vi "Annotate April.vi"(6 "hilight":bool, 7 "Annotate":bool, 9 "cutoffs":T1, 10 "Detected Tags":T3(array[cluster]), 11 "Refnum in":T2) -> (1 "margins":dbl[](array[numeric]), 2 "tags":T3(array[cluster]), 3 "Refnum out":T2)   [LabVIEW 2023]
uses:
  <vilib>/vision/Image Controls.llb/IMAQ Image.ctl
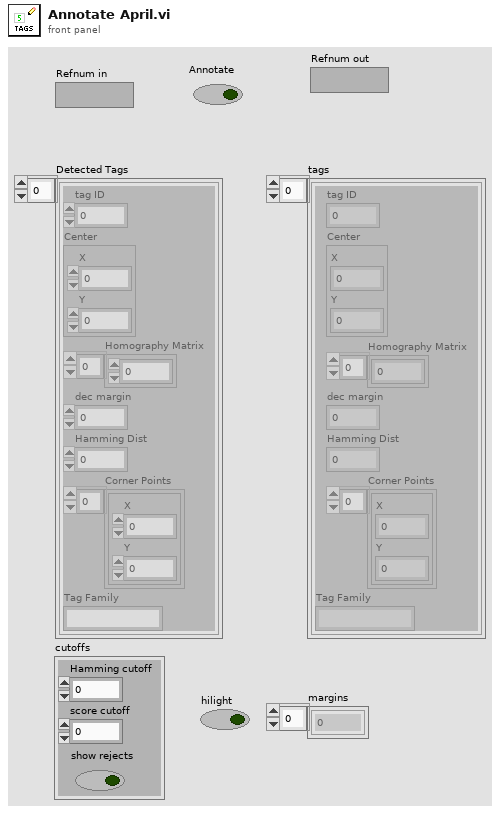
[diagram p1: front panel]
types:
  T1 = cluster{"Hamming cutoff":i32, "score cutoff":dbl, "show rejects":bool}
  T2 = typedef "IMAQ Image.ctl" = refnum<image>
  T3 = cluster{"tag ID":i32, "Center":cluster{"X":dbl, "Y":dbl}, "Homography Matrix":dbl[], "dec margin":dbl, "Hamming Dist":i32, "Corner Points":cluster{"X":dbl, "Y":dbl}[], "Tag Family":string}[]
  T4 = cluster{"Desired Font (Application)":enum16{"User-specified Font", "Application Font", "System Font", "Dialog Font"}, "[User-specified Font]":cluster{"Font Name":string, "Size":i16, "Strikeout?":bool, "Italic?":bool, "Underline?":bool, "Outline?":bool, "Shadow?":bool, "Bold?":bool, "Rotation Angle":dbl}, "Horizontal Alignment":i16, "Vertical Alignment":i16}
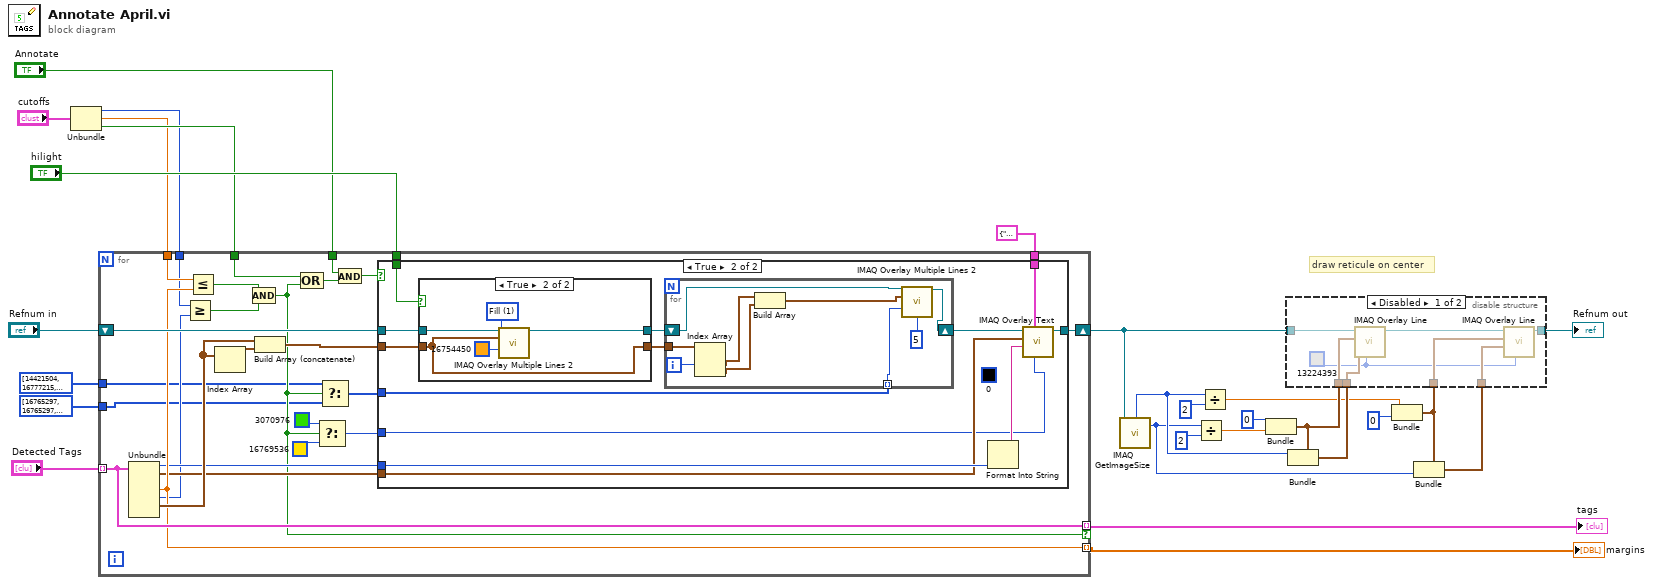
[diagram p0: block diagram]
diagram:
  # "draw reticule on center"
  n1 = Unbundle("cutoffs") -> ("Hamming cutoff"=w4:i32, "score cutoff"=w5:dbl, "show rejects"=w6:bool)
  n2 = for {
    tunnel: "Detected Tags" -> [w51] mode=indexing
    shift-right: [w53] -> w22
    shift-left: "Refnum in" -> [w54]
    tunnel: [w51] -> w27 mode=indexing if=w32
    tunnel: [w50] -> w25 mode=indexing
    tunnel: w6 -> [w42]
    tunnel: T4 {"Desired Font (Application)"=enum."Application Font", "[User-specified Font]"={"Font Name"="", "Size"=12, "Strikeout?"=FALSE, "Italic?"=FALSE, "Underline?"=FALSE, "Outline?"=FALSE, "Shadow?"=FALSE, "Bold?"=FALSE, "Rotation Angle"=0.0}, "Horizontal Alignment"=1, "Vertical Alignment"=2} ("Font, Size & Style") -> [w39]
    tunnel: "hilight" -> [w38]
    tunnel: w5 -> [w37]
    tunnel: w4 -> [w35]
    tunnel: u32[] [14421504, 16777215, 16777215, 3070976] -> [w31]
    tunnel: u32[] [16765297, 16765297, 16765297, 16765297] -> [w30]
    tunnel: "Annotate" -> [w28]
    n3 = Unbundle(w51) -> ("tag ID"=w49:i32, "Center"=w48:cluster{"X":dbl, "Y":dbl}, "dec margin"=w50:dbl, "Hamming Dist"=w36:i32, "Corner Points"=w52:cluster{"X":dbl, "Y":dbl}[])  [unwired: 2 out]
    n4 = Greater Or Equal?(x=w35, y=w36) -> (x >= y?=w33:bool)
    n5 = Less Or Equal?(x=w37, y=w50) -> (x <= y?=w34:bool)
    n6 = Index Array(array=w52) -> (element=w44:cluster{"X":dbl, "Y":dbl})  [unwired: 1 in]
    n7 = Compound Arithmetic op=AND(w34, w33) -> (w32:bool)
    n8 = Build Array (concatenate)(w52, w44) -> (w43:cluster{"X":dbl, "Y":dbl}[])
    n9 = Compound Arithmetic op=OR(w42, w32) -> (w41:bool)
    n10 = Select(t=u32 3070976 ("Color"), s=w32, f=u32 16769536 ("Color")) -> (s? t:f=w45:u32)
    n11 = Select(t=w31, s=w32, f=w30) -> (s? t:f=w40:u32[])
    n12 = And(x=w28, y=w41) -> (x .and. y?=w29:bool)
    n13 = case shown="True" w29 {
      tunnel: w54 -> [w55 w59]
      tunnel: [w55 w68] -> w53
      tunnel: w49 -> [_ w67]
      tunnel: w48 -> [_ w66]
      tunnel: w45 -> [_ w62]
      tunnel: w43 -> [_ w60]
      tunnel: w40 -> [_ w64]
      tunnel: w39 -> [_ w63]
      tunnel: w38 -> [_ w56]
      frame False {
      }
      frame True {
        (unwired) u32 0 ("Color")
        n14 = case shown="True" w56 {
          tunnel: w60 -> [w69 w72]
          tunnel: w59 -> [w70 w74]
          tunnel: [w70 w75] -> w58
          tunnel: [w69 w72] -> w57
          frame False {
          }
          frame True {
            w71 = u32 1 items=["Frame", "Fill"] ("Drawing Mode (Frame)")
            n15 = call "IMAQ Overlay Multiple Lines 2"("Image"=w74, "Line End Points"=w72, "Drawing Mode (Frame)"=w71, "Color"=u32 16754450) -> ("Image Out"=w75:T2)  [unwired: 10 in, 1 out]
          }
        }
        n16 = for {
          shift-right: [w80] -> w61
          shift-left: w58 -> [w79]
          tunnel: w57 -> [w84]
          tunnel: w64 -> [w76] mode=indexing
          i -> [w83]
          n17 = Index Array(array=w84, index #1=w83) -> (element #1=w81:cluster{"X":dbl, "Y":dbl}, element #2=w78:cluster{"X":dbl, "Y":dbl})  [unwired: 1 in]
          n18 = Build Array(w81, w78) -> (w82:cluster{"X":dbl, "Y":dbl}[])
          n19 = call "IMAQ Overlay Multiple Lines 2"("Image"=w79, "Line End Points"=w82, "Color"=w76, "Width"=u32 5) -> ("Image Out"=w80:T2)  [unwired: 10 in, 1 out]
        }
        n20 = Format Into String(w67) -> (resulting string=w65:string)  [unwired: 3 in, 1 out]
        n21 = call "IMAQ Overlay Text"("Text Color (black)"=w62, "Font, Size & Style"=w63, "String"=w65, "Origin"=w66, "Image"=w61) -> ("Image Out"=w68:T2)  [unwired: 5 in, 1 out]
      }
    }
  }
  "tags" <- w27
  "margins" <- w25
  n22 = call "IMAQ GetImageSize"("Image"=w22) -> ("Y Resolution"=w12:i32, "X Resolution"=w17:i32)  [unwired: 3 in, 1 out]
  n23 = Divide(x=w12, y=2 ("X")) -> (x/y=w19:dbl)
  n24 = Divide(x=w17, y=2 ("X")) -> (x/y=w13:dbl)
  n25 = Bundle("X"=0, w19) -> (w18:cluster{"X":i32, dbl})  [unwired: 1 in]
  n26 = Bundle(cluster=w18, "X"=w17) -> (w16:cluster{"X":i32, dbl})  [unwired: 1 in]
  n27 = Bundle(w13, "X"=0) -> (w10:cluster{dbl, "X":i32})  [unwired: 1 in]
  n28 = Bundle(cluster=w10, "X"=w12) -> (w11:cluster{dbl, "X":i32})  [unwired: 1 in]
  n29 = disable-structure shown="Disabled" {
    disable-tunnel: [w91 w93] -> w23
    disable-tunnel: w22 -> [w90 w93]
    disable-tunnel: w18 -> [w89 _]
    disable-tunnel: w16 -> [w88 _]
    disable-tunnel: w11 -> [w87 _]
    disable-tunnel: w10 -> [w86 _]
    frame Disabled {
      w85 = u32 13224393 ("Color")
      n30 = call "IMAQ Overlay Line"("Color"=w85, "End Point"=w88, "Start Point"=w89, "Image"=w90) -> ("Image Out"=w92:T2)  [unwired: 6 in, 1 out]
      n31 = call "IMAQ Overlay Line"("Color"=w85, "End Point"=w87, "Start Point"=w86, "Image"=w92) -> ("Image Out"=w91:T2)  [unwired: 6 in, 1 out]
    }
    frame Enabled {
    }
  }
  "Refnum out" <- w23
